vi "Draw PCBS.vi"(0 "data in":T6, 1 "XY Graph":refnum<vi>, 7 "PCB List":T5(array[cluster]), 11 "error in (no error)":errorcluster, 13 "Diagnostic Station PCB":T1) -> (4 "PCB Outlines":T14(array[cluster]), 10 "Plot colours[]":u32[](array[colorbox]), 15 "error out":errorcluster)   [LabVIEW 2013, in "Manipulate IPF.lvlib"]
uses:
  Manipulate IPF.lvlib
  3013/code/Modules/GUI/GUI_5/subPanels/edit/type_def/data.ctl
  3013/code/Modules/Configuration/type_def/Scan Params.ctl
  3013/code/Modules/Configuration/type_def/Profile Resolution.ctl
  3013/code/Modules/Preprocess Data/type_def/direction.ctl
  3013/code/Modules/Inspection/Data/Panel_class/type_def/Config File data.ctl
  3013/code/Modules/Inspection/type_def/Pos and Rot.ctl
  3013/code/Modules/Inspection/Data/PCB_class/type_def/PCB Params.ctl
  3013/code/Modules/Inspection/Data/Panel_class/type_def/BarCode Params.ctl
  3013/code/Modules/Barcode Reader/type_def/id.ctl
  3013/code/Modules/Inspection/Data/Panel_class/type_def/inspection data.ctl
  3013/code/Modules/Inspection/type_def/Range Limits.ctl
  Mike/APG_mike a3Di.lvlib
  <vilib>/Analysis/NI_AALBase.lvlib
  3013/code/Modules/Inspection/Inspection.lvlib
  3014/code/modules/Results DB/Results DB.lvlib
  3013/code/Modules/Inspection/Data/PCB_class/PCB.lvclass
  3013/code/Modules/Barcode Reader/Barcode Reader.lvlib
  3013/code/Modules/Inspection/Data/Panel_class/Panel.lvclass
  3013/code/Modules/Configuration/Config.lvlib
  3013/code/Modules/Preprocess Data/PreProcess.lvlib
  3013/code/Modules/GUI/GUI_5/subPanels/edit/edit.lvlib
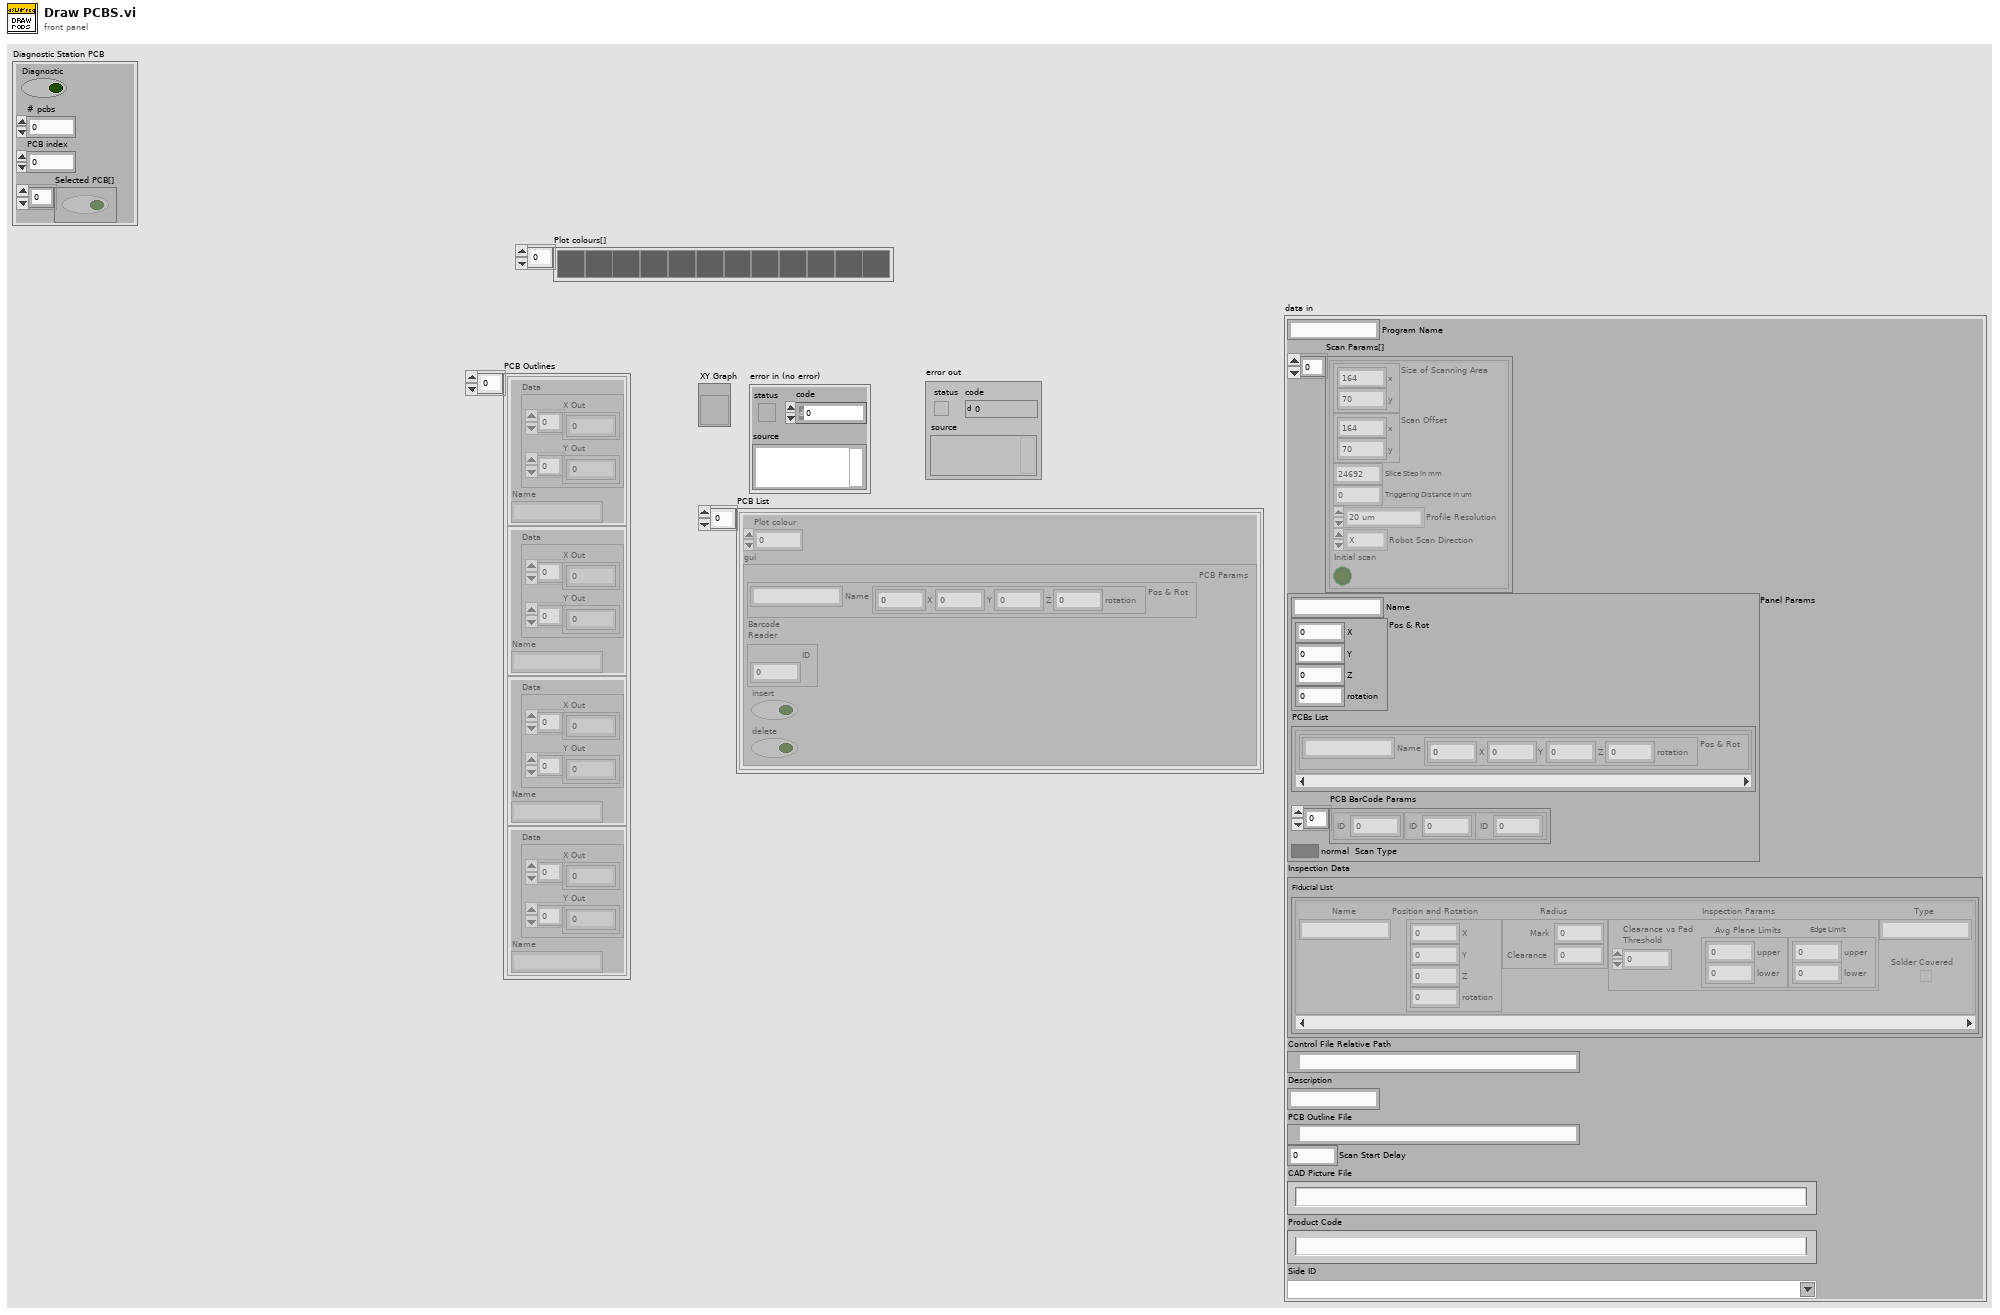
[diagram p1: front panel]
types:
  T1 = cluster{"Diagnostic":bool, "# pcbs":u32, "PCB index":u32, "Selected PCB[]":bool[]}
  T2 = typedef "Inspection.lvlib/PCB.lvclass/PCB Params.ctl" = cluster{"Name":string, "Pos & Rot":T3}
  T3 = typedef "Inspection.lvlib/Pos and Rot.ctl" = cluster{"X":dbl, "Y":dbl, "Z":dbl, "rotation":dbl}
  T4 = typedef "Barcode Reader.lvlib/id.ctl" = u8
  T5 = cluster{"Plot colour":u32, "gui":cluster{"PCB Params":T2, "Barcode\nReader":cluster{"ID":T4}, "insert":bool, "delete":bool}}[]
  T6 = typedef "GUI.lvlib/subPanel.lvlib/edit.lvlib/data.ctl" = cluster{"Program Name":string, "Scan Params[]":T7[], "Panel Params":T10, "Inspection Data":T12, "Control File Relative Path":path, "Description":string, "PCB Outline File":path, "Scan Start Delay":dbl, "CAD Picture File":string, "Product Code":string, "Side ID":string}
  T7 = typedef "Config.lvlib/Scan Params.ctl" = cluster{"Size of Scanning Area":cluster{"x":dbl, "y":dbl}, "Scan Offset":cluster{"x":dbl, "y":dbl}, "Slice Step in mm":dbl, "Triggering Distance in mm":dbl, "Triggering Distance in um":dbl, "Profile Resolution":T8, "Version":string, "Robot Scan Direction":T9, "Initial scan":bool}
  T8 = typedef "Config.lvlib/Profile Resolution.ctl" = enum8{"20 um", "40 um"}
  T9 = typedef "PreProcess.lvlib/direction.ctl" = enum8{"X", "Y"}
  T10 = typedef "Inspection.lvlib/Panel.lvclass/Config File data.ctl" = cluster{"Name":string, "Pos & Rot":T3, "PCBs List":cluster{"PCB Params":T2}[], "PCB BarCode Params":T11[], "Scan Type":bool}
  T11 = typedef "Inspection.lvlib/Panel.lvclass/BarCode Params.ctl" = cluster{"ID":T4}
  T12 = typedef "Inspection.lvlib/Panel.lvclass/inspection data.ctl" = cluster{"Fiducial List":cluster{"Name":string, "Position and Rotation":T3, "Radius":cluster{"Mark":dbl, "Clearance":dbl}, "Inspection Params":cluster{"Clearance vs Pad\nThreshold":dbl, "Avg Plane Limits":T13, "Edge Limit":T13}, "Type":string, "Solder Covered":bool}[]}
  T13 = typedef "Inspection.lvlib/Range Limits.ctl" = cluster{"upper":sgl, "lower":sgl}
  T14 = cluster{"Data":cluster{"X Out":dbl[], "Y Out":dbl[]}, "Name":string}[]
  T15 = cluster{"ODB2CPF.exe":path, "TCFToArtworkCPF.exe":path, "TCFToCPFLabels.exe":path, "7z.exe":path, "UpdateTCFLibrary.exe":path, "a3DiPackageTests":path, "Error Codes":path, "TCFToCuboidRefCPF":path, "TCFToArtworkRefCPF":path, "ExtractPKG":path, "ExtractTCFFromODBFileForPKG":path, "OutLineFilterTCFPKG":path, "GenerateLibraryFromTCF":path, "FlipCPF":path, "FlipTCF":path, "TCFToJointBridgeCPF":path, "TCFToJointFR4CPF":path}
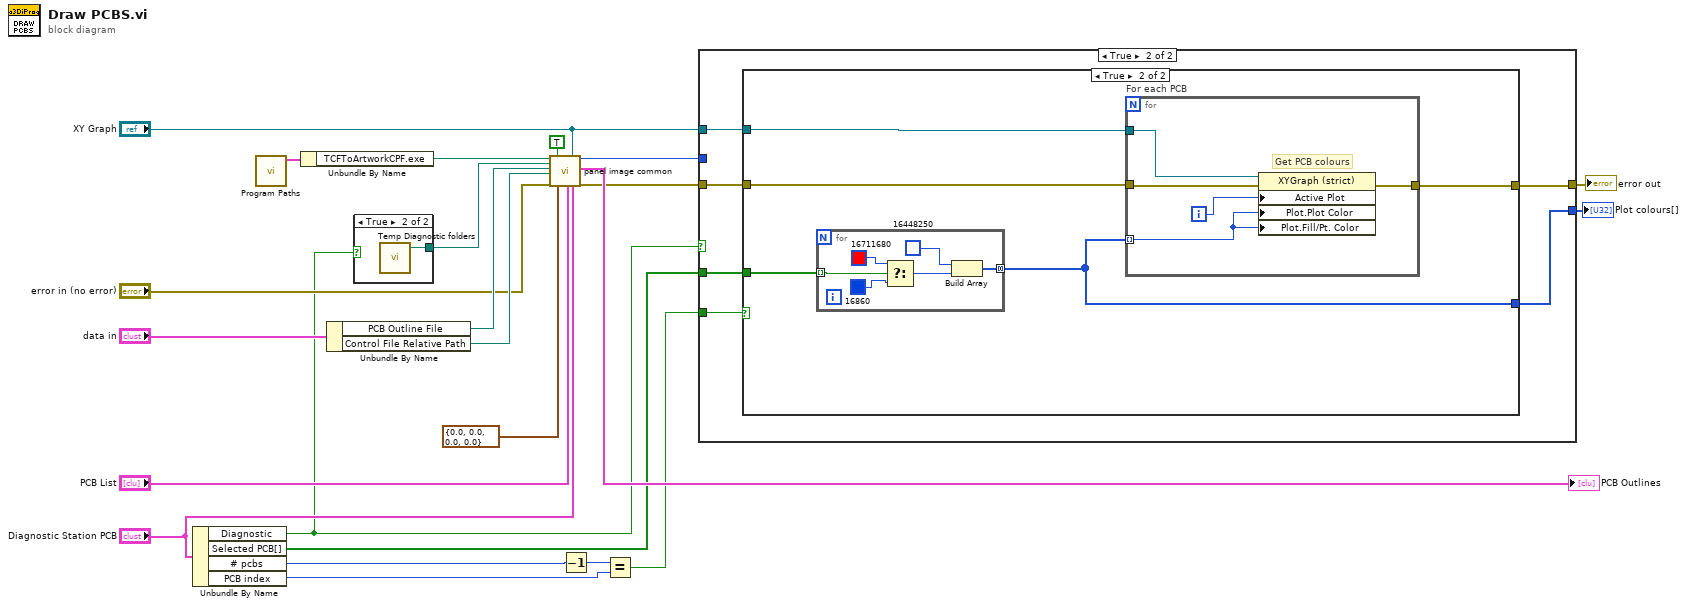
[diagram p0: block diagram]
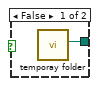
[diagram p2: hidden frame]
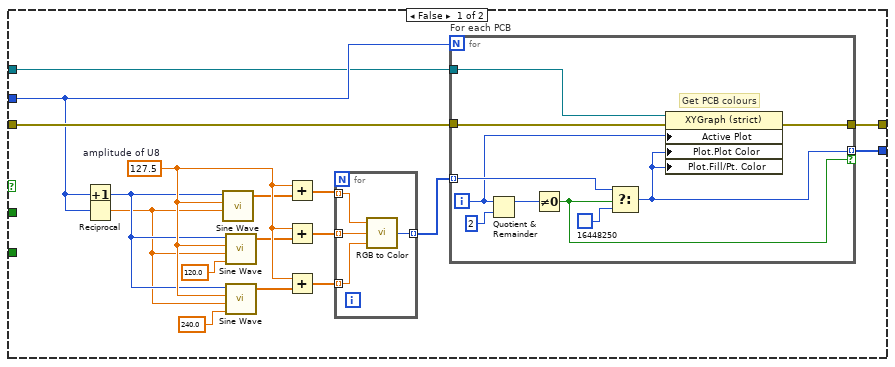
[diagram p3: hidden frame]
diagram:
  n1 = Unbundle By Name("Diagnostic Station PCB") -> ("Diagnostic"=w1:bool, "Selected PCB[]"=w7:bool[], "# pcbs"=w4:u32, "PCB index"=w3:u32)
  n2 = call "Program Paths.vi"() -> ("Program paths"=w21:T15)  [unwired: 10 in]
  n3 = Unbundle By Name(w21) -> ("TCFToArtworkCPF.exe"=w20:path)
  n4 = Unbundle By Name("data in") -> ("PCB Outline File"=w18:path, "Control File Relative Path"=w17:path)
  n5 = case shown="True" w1 {
    tunnel: [w24 w25] -> w19
    frame False {
      n6 = call "temporay folder.vi"() -> ("temporay folder"=w24:path)  [unwired: 11 in]
    }
    frame True {
      n7 = call "Temp Diagnostic folders.vi"() -> ("Diag temp folder"=w25:path)  [unwired: 14 in, 1 out]
    }
  }
  n8 = call "panel image common.vi"("TCFToArtworkCPF.exe"=w20, "temporary folder"=w19, "PCB Outline File"=w18, "Control File Relative Path"=w17, "error in (no error)"="error in (no error)", "APG"=TRUE, "Panel Pos & Rot"=T3 {"X"=0.0, "Y"=0.0, "Z"=0.0, "rotation"=0.0}, "PCB List"="PCB List", "XY Graph"="XY Graph", "Diagnostic Station PCB"="Diagnostic Station PCB") -> ("# plots"=w13:i32, "PCB Outlines[]"=→"PCB Outlines":T14, "error out"=w14:errorcluster)  [unwired: 7 in]
  n9 = Decrement(x=w4) -> (x-1=w5:u32)
  n10 = Equal?(x=w5, y=w3) -> (x = y?=w2:bool)
  n11 = case shown="True" w1 {
    tunnel: [w42 w58] -> w23
    tunnel: w14 -> [w40 w60]
    tunnel: w13 -> [w39 _]
    tunnel: "XY Graph" -> [w38 w61]
    tunnel: w7 -> [_ w62]
    tunnel: [w26 w59] -> w6
    tunnel: w2 -> [_ w57]
    frame False {
      w37 = 127.5  # amplitude of U8
      n12 = Increment(x=w39) -> (x+1=w36:i32)
      n13 = Reciprocal(x=w39) -> (1/x=w35:dbl)
      n14 = call <vilib>:"Sine Wave.vi"("samples"=w36, "amplitude"=w37, "frequency"=w35) -> ("sine wave"=w34:dbl[])  [unwired: 2 in, 2 out]
      n15 = call <vilib>:"Sine Wave.vi"("samples"=w36, "amplitude"=w37, "frequency"=w35, "phase in"=120.0) -> ("sine wave"=w30:dbl[])  [unwired: 1 in, 2 out]
      n16 = call <vilib>:"Sine Wave.vi"("samples"=w36, "amplitude"=w37, "frequency"=w35, "phase in"=240.0) -> ("sine wave"=w29:dbl[])  [unwired: 1 in, 2 out]
      n17 = Add(x=w37, y=w34) -> (x+y=w31:dbl[])
      n18 = Add(x=w37, y=w30) -> (x+y=w32:dbl[])
      n19 = Add(x=w37, y=w29) -> (x+y=w33:dbl[])
      n20 = for {
        tunnel: w31 -> [w45] mode=indexing
        tunnel: w32 -> [w44] mode=indexing
        tunnel: w33 -> [w46] mode=indexing
        tunnel: [w43] -> w41 mode=indexing
        n21 = call <vilib>:"RGB to Color.vi"("B"=w46, "G"=w44, "R"=w45) -> ("Color"=w43:u32)
      }
      n22 = for "For each PCB" {
        N: w39 -> [_]
        tunnel: w38 -> [w52]
        tunnel: w40 -> [w53]
        tunnel: [w54] -> w42 mode=indexing if=w47
        tunnel: w41 -> [w51] mode=indexing
        tunnel: [w49] -> w26
        i -> [w48]
        # "Get PCB colours"
        n23 = Quotient & Remainder(x=w48, y=2) -> (x-y*floor(x/y)=w55:i32)  [unwired: 1 out]
        n24 = Not Equal To 0?(x=w55) -> (x != 0?=w47:bool)
        n25 = Select(t=w51, s=w47, f=u32 16448250) -> (s? t:f=w54:u32)
        n26 = property on="Property Node" class="XYGraph (strict)"(reference=w52, error in=w53, "Active Plot"=w48, "Plot.Plot Color"=w54, "Plot.Fill/Pt. Color"=w54) -> (error out=w49:errorcluster)  [unwired: 1 out]
      }
    }
    frame True {
      n27 = case shown="True" w57 {
        tunnel: w62 -> [_ w68]
        tunnel: w61 -> [_ w67]
        tunnel: w60 -> [w63 w66]
        tunnel: [w63 w65] -> w59
        tunnel: [_ w64] -> w58
        frame False {
        }
        frame True {
          n28 = for {
            tunnel: [w76] -> w64 mode=concatenating
            tunnel: w68 -> [w77] mode=indexing
            n29 = Select(t=u32 16711680, s=w77, f=u32 16860) -> (s? t:f=w75:u32)
            n30 = Build Array(u32 16448250, w75) -> (w76:u32[])
          }
          n31 = for "For each PCB" {
            tunnel: w67 -> [w72]
            tunnel: w66 -> [w73]
            tunnel: w64 -> [w69] mode=indexing
            tunnel: [w71] -> w65
            i -> [w70]
            # "Get PCB colours"
            n32 = property on="Property Node" class="XYGraph (strict)"(reference=w72, error in=w73, "Active Plot"=w70, "Plot.Plot Color"=w69, "Plot.Fill/Pt. Color"=w69) -> (error out=w71:errorcluster)  [unwired: 1 out]
          }
        }
      }
    }
  }
  "Plot colours[]" <- w23
  "error out" <- w6
